vi "ext_trig_counter.vi"() -> ()   [LabVIEW 2016, in "Utilities.lvlib" / "_TEST.lvlib"]
uses:
  _TEST.lvlib
  Drivers/C8855-01/Trigger Mode.ctl
  Drivers/C8855-01/Transfer Mode.ctl
  <vilib>/DAQmx/create/channels.llb/DAQmx Create Channel (CO-Pulse Generation-Time).vi
  <vilib>/DAQmx/configure/timing.llb/DAQmx Timing (Implicit).vi
  Drivers/C8855-01/C8855-01.lvlib
panel:
  out "Elapsed (ms)":dbl format="%#.6g"
  out "Data":u16[](graph)
  in  "Initial Delay (s)":dbl=5.0 format="%#_13g"
  out "Photon Counter ID":u8
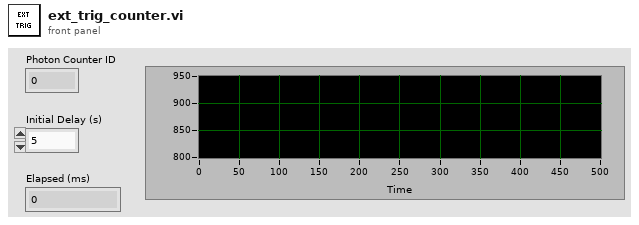
[diagram p1: front panel]
types:
  T1 = typedef "Drivers.lvlib/C8855-01.lvlib/Transfer Mode.ctl" = u8
  T2 = typedef "Drivers.lvlib/C8855-01.lvlib/Trigger Mode.ctl" = u8
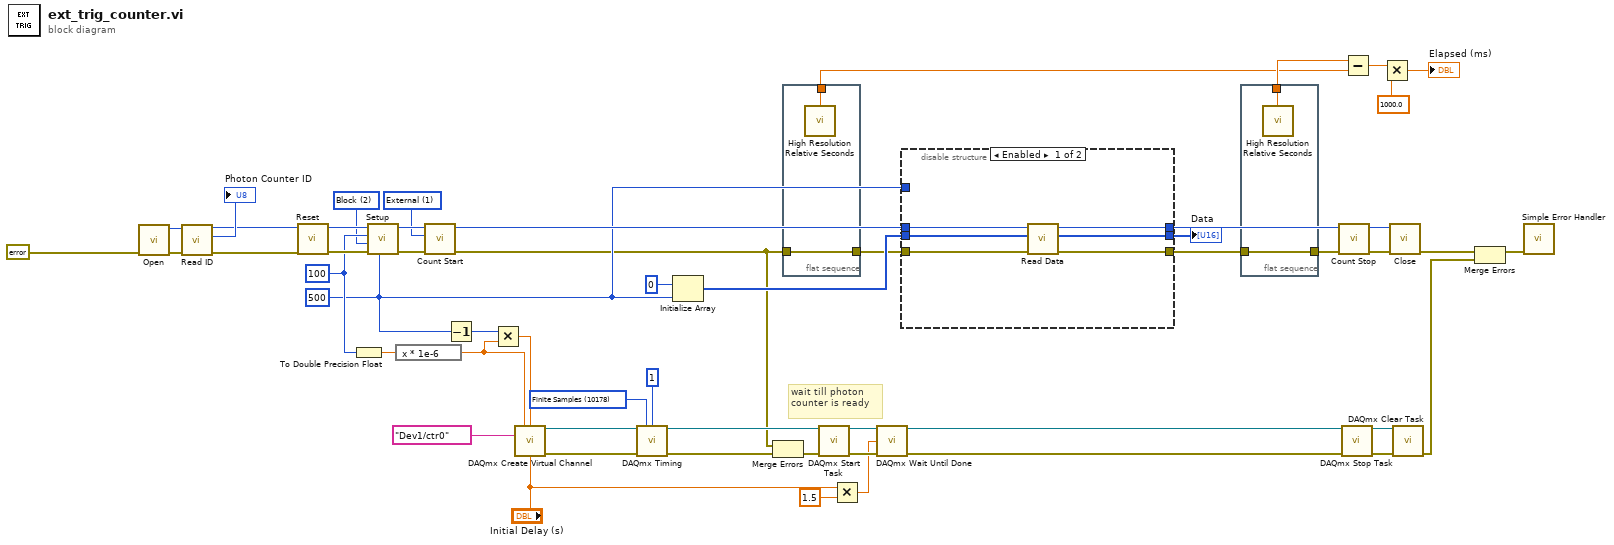
[diagram p0: block diagram]
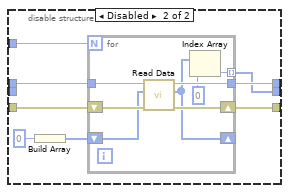
[diagram p2: hidden frame]
diagram:
  w22 = T1 2 items=["Single"=1, "Block"=2] ("Transfer Mode")
  w29 = 10178 items=["Finite Samples"=10178, "Continuous Samples"=10123, "Hardware Timed Single Point"=12522] ("sample mode")
  w10 = 500 ("Number of Gate")
  w36 = u32 100 ("Gate Time (us)")
  w44 = T2 1 items=["Software", "External"] ("Trigger Mode")
  # "wait till photon counter is ready"
  n1 = call "Open.vi"("error in (no error)"=errorcluster {"status"=FALSE, "code"=0, "source"=""}) -> ("error out"=w52:errorcluster, "Handle"=w53:u32)  [unwired: 9 in]
  n2 = call "Read ID.vi"("error in (no error)"=w52, "handle in"=w53) -> ("error out"=w50:errorcluster, "ID"=→"Photon Counter ID":u8, "handle out"=w49:u32)  [unwired: 7 in]
  n3 = call "Reset.vi"("error in (no error)"=w50, "handle in"=w49) -> ("error out"=w48:errorcluster, "handle out"=w45:u32)  [unwired: 8 in]
  n4 = To Double Precision Float(number=w36) -> (double precision float=w35:dbl)
  n5 = call "Setup.vi"("Number of Gate"=w10, "error in (no error)"=w48, "Transfer Mode"=w22, "Gate Time (us)"=w36, "Handle"=w45) -> ("error out"=w47:errorcluster, "Handle out"=w46:u32)  [unwired: 5 in]
  n6 = expression code="x * 1e-6"(w35) -> (w30:dbl)
  n7 = call "Count Start.vi"("error in (no error)"=w47, "Trigger Mode"=w44, "handle in"=w46) -> ("error out"=w8:errorcluster, "handle out"=w42:u32)  [unwired: 7 in]
  n8 = Decrement(x=w10) -> (x-1=w34:i32)
  n9 = Multiply(x=w34, y=w30) -> (x*y=w33:dbl)
  n10 = call-poly <vilib>:"DAQmx Create Virtual Channel.vi"("high time"=w30, "low time"=w33, "counter"=tag "Dev1/ctr0" ("physical channels"), "initial delay"="Initial Delay (s)") -> ("task out"=w32:refnum<k21>, "error out"=w31:errorcluster)  [unwired: 10 in]
  n11 = call-poly <vilib>:"DAQmx Timing.vi"("task/channels in"=w32, "sample mode"=w29, "samples per channel"=1, "error in"=w31) -> ("task out"=w28:refnum<k21>, "error out"=w15:errorcluster)  [unwired: 10 in]
  n12 = Initialize Array(u16 0 ("element"), w10) -> (w41:u16[])
  n13 = Merge Errors(w8, w15) -> (w14:errorcluster)
  n14 = flat-sequence {
    tunnel: [w56] -> w9
    tunnel: w8 -> [w56]
    tunnel: [w55] -> w4
    frame #0 {
      n15 = call <vilib>:"High Resolution Relative Seconds.vi"() -> ("relative seconds"=w55:dbl)
    }
  }
  n16 = call <vilib>:"DAQmx Start Task.vi"("task/channels in"=w28, "error in"=w14) -> ("task out"=w27:refnum<k21>, "error out"=w26:errorcluster)  [unwired: 12 in]
  n17 = Multiply(x="Initial Delay (s)", y=1.5) -> (x*y=w11:dbl)
  n18 = call <vilib>:"DAQmx Wait Until Done.vi"("task/channels in"=w27, "timeout (sec)"=w11, "error in"=w26) -> ("task out"=w18:refnum<k21>, "error out"=w20:errorcluster)  [unwired: 11 in]
  n19 = disable-structure shown="Enabled" {
    disable-tunnel: w42 -> [w62 w69]
    disable-tunnel: w41 -> [w61 _]
    disable-tunnel: [w60 w64] -> w40
    disable-tunnel: [w59 w63] -> w21
    disable-tunnel: [w58 w67] -> w6
    disable-tunnel: w9 -> [w57 w68]
    disable-tunnel: w10 -> [_ w70]
    frame Enabled {
      n20 = call "Read Data.vi"("error in (no error)"=w57, "buffer in"=w61, "handle in"=w62) -> ("error out"=w58:errorcluster, "buffer out"=w59:u16[], "handle out"=w60:u32)  [unwired: 6 in]
    }
    frame Disabled {
      n21 = Build Array(u16 0 ("element")) -> (w65:u16[])
      n22 = for {
        N: w70 -> [_]
        tunnel: w69 -> [w78]
        shift-right: [w76] -> w67
        shift-left: w68 -> [w77]
        shift-right: [w73] -> _
        shift-left: w65 -> [w75]
        tunnel: [w74] -> w64
        tunnel: [w71] -> w63 mode=indexing
        n23 = call "Read Data.vi"("error in (no error)"=w77, "buffer in"=w75, "handle in"=w78) -> ("error out"=w76:errorcluster, "buffer out"=w73:u16[], "handle out"=w74:u32)  [unwired: 6 in]
        n24 = Index Array(array=w73, index=0) -> (element=w71:u16)
      }
    }
  }
  "Data" <- w21
  n25 = flat-sequence {
    tunnel: [w80] -> w7
    tunnel: w6 -> [w80]
    tunnel: [w79] -> w5
    frame #0 {
      n26 = call <vilib>:"High Resolution Relative Seconds.vi"() -> ("relative seconds"=w79:dbl)
    }
  }
  n27 = call "Count Stop.vi"("error in (no error)"=w7, "handle in"=w40) -> ("error out"=w38:errorcluster, "handle out"=w39:u32)  [unwired: 8 in]
  n28 = call <vilib>:"DAQmx Stop Task.vi"("task/channels in"=w18, "error in"=w20) -> ("task out"=w17:refnum<k21>, "error out"=w19:errorcluster)  [unwired: 12 in]
  n29 = Subtract(x=w5, y=w4) -> (x-y=w3:dbl)
  n30 = Multiply(x=w3, y=1000.0) -> (x*y=→"Elapsed (ms)":dbl)
  n31 = call "Close.vi"("error in (no error)"=w38, "handle in"=w39) -> ("error out"=w25:errorcluster)  [unwired: 9 in]
  n32 = call <vilib>:"DAQmx Clear Task.vi"("task in"=w17, "error in"=w19) -> ("error out"=w23:errorcluster)  [unwired: 13 in]
  n33 = Merge Errors(w25, w23) -> (w24:errorcluster)
  n34 = call <vilib>:"Simple Error Handler.vi"("error in (no error)"=w24) -> ()  [unwired: 4 in, 5 out]
